vi "Read Log Messages.vi"(8 "error in (no error)":errorcluster, 11 "Test System in":refnum<class "Test System.lvclass">) -> (0 "error out":errorcluster, 2 "Log Messages":string[](array[string]), 3 "Test System out":refnum<class "Test System.lvclass">)   [LabVIEW 2021, in "Test System.lvclass"]
uses:
  Test System.lvclass
  Test System.lvclass/Test System.ctl
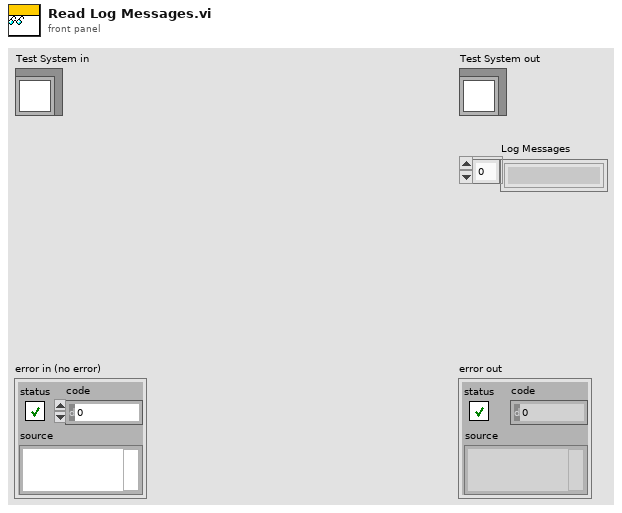
[diagram p1: front panel]
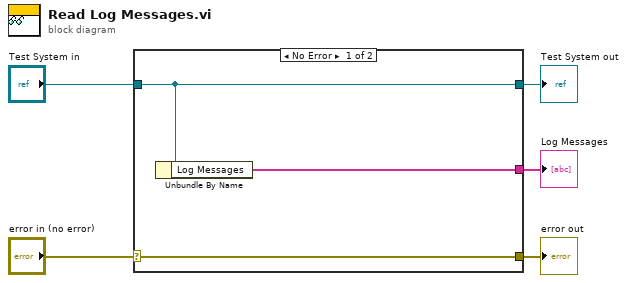
[diagram p0: block diagram]
diagram:
  n1 = case shown="No Error" "error in (no error)" {
    selector: "error in (no error)" -> [w8 w9]
    tunnel: [w8 w9] -> w4
    tunnel: [w7 w10] -> w2
    tunnel: "Test System in" -> [w7 w10]
    tunnel: [w6 _] -> w1
    frame No Error {
      n2 = Unbundle By Name(w7) -> ("Log Messages"=w6:string[])
    }
    frame Error {
    }
  }
  "error out" <- w4
  "Test System out" <- w2
  "Log Messages" <- w1
